vi "Run.vi"(8 "error in (no error)":errorcluster caption="entrée d'erreur (pas d'erreur)", 9 "labels":string[][](array[string]), 10 "X":string[][](array[string]), 11 "Silhouette_Samples.lvclass":refnum<class "Silhouette_Samples.lvclass">) -> (0 "error out":errorcluster caption="sortie d'erreur", 2 "Data":T1, 3 "Silhouette_Samples.lvclass":refnum<class "Silhouette_Samples.lvclass">)   [LabVIEW 2020, in "Silhouette_Samples.lvclass"]
doc: "Returns : \n\n- silhouette : array, shape = [n_samples]\nSilhouette Coefficient for each samples."
uses:
  Silhouette_Samples.lvclass
  Silhouette_Samples.lvclass/Silhouette_Samples.ctl
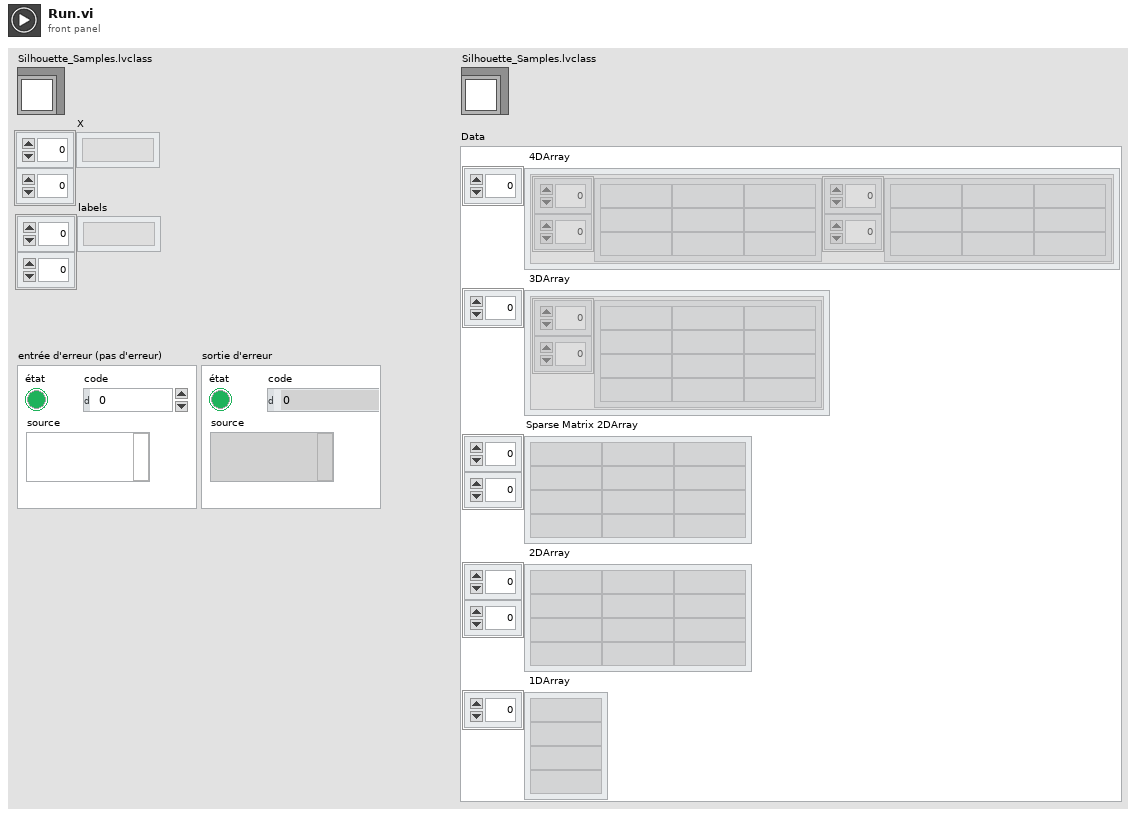
[diagram p1: front panel]
types:
  T1 = cluster{" 4DArray":cluster{"1":string[][], "2":string[][]}[], " 3DArray":cluster{"Tableau":string[][]}[], "Sparse Matrix 2DArray":string[][], " 2DArray":string[][], " 1DArray":string[]}
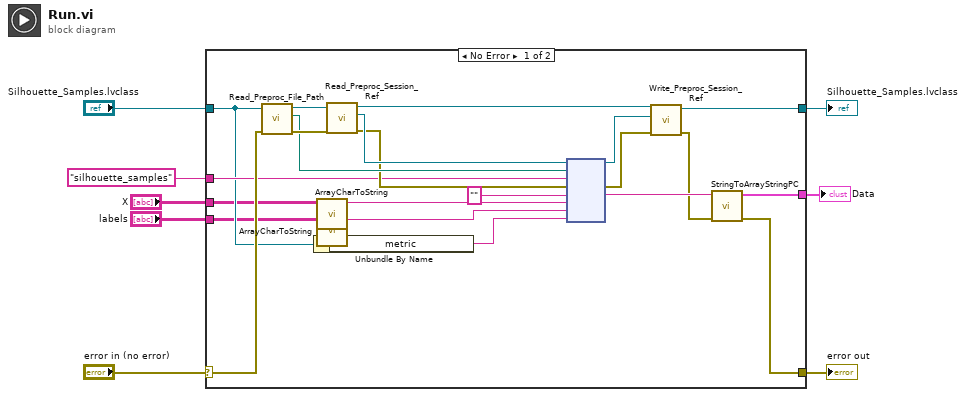
[diagram p0: block diagram]
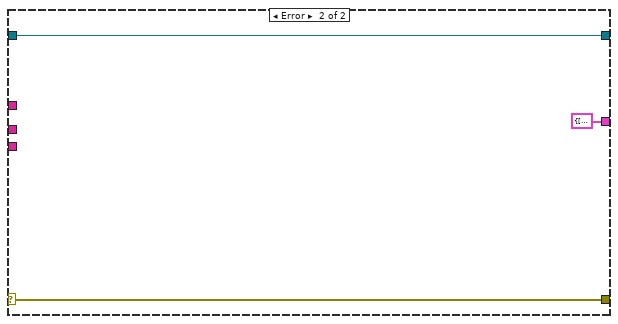
[diagram p2: hidden frame]
diagram:
  n1 = case shown="No Error" "error in (no error)" {
    selector: "error in (no error)" -> [w21 w33]
    tunnel: [w10 w33] -> w7
    tunnel: [w13 w32] -> w5
    tunnel: "Silhouette_Samples.lvclass" -> [w19 w32]
    tunnel: "silhouette_samples" -> [w20 _]
    tunnel: "X" -> [w17 _]
    tunnel: "labels" -> [w16 _]
    tunnel: [w9 T1 {" 4DArray"=[], " 3DArray"=[], "Sparse Matrix 2DArray"=[], " 2DArray"=[], " 1DArray"=[]} ("Data")] -> w1
    frame No Error {
      n2 = call-dynamic "Read_Preproc_File_Path.vi"("error in (no error)"=w21, "Python in"=w19) -> ("error out"=w29:errorcluster, "File_Path"=w28:path, "Python out"=w30:refnum<class "Silhouette_Samples.lvclass">)  [unwired: 7 in]
      n3 = Unbundle By Name(w19) -> ("metric"=w18:string)
      n4 = call "ArrayCharToString.vi"("TAB"=w17) -> ("Instruction"=w15:string)  [unwired: 10 in]
      n5 = call "ArrayCharToString.vi"("TAB"=w16) -> ("Instruction"=w14:string)  [unwired: 10 in]
      n6 = call-dynamic "Read_Preproc_Session_Ref.vi"("error in (no error)"=w29, "Python in"=w30) -> ("error out"=w26:errorcluster, "Session_ref"=w27:refnum<k35>, "Python out"=w25:refnum<class "Silhouette_Samples.lvclass">)  [unwired: 7 in]
      n7 = node(w27, w28, w20, w26, "", w15, w14, w18) -> (w23:refnum<k35>, w24:errorcluster, w12:string)  [unwired: 3 in, 2 out]
      n8 = call-dynamic "Write_Preproc_Session_Ref.vi"("error in (no error)"=w24, "Session_ref"=w23, "Python in"=w25) -> ("error out"=w11:errorcluster, "Python out"=w13:refnum<class "Silhouette_Samples.lvclass">)  [unwired: 7 in]
      n9 = call "StringToArrayStringPC.vi"("sortie d'erreur"=w11, "Return value"=w12) -> ("sortie d'erreur"=w10:errorcluster, "Data"=w9:T1)  [unwired: 8 in]
    }
    frame Error {
    }
  }
  "error out" <- w7
  "Silhouette_Samples.lvclass" <- w5
  "Data" <- w1
